vi "Gyro Global.vi"() -> ()   [LabVIEW 2014]
panel:
  in  "Boolean":bool
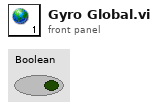
[diagram p1: front panel]
diagram:
